vi "6500电流加载及换向回读.vi"(0 "2700 in":refnum<visa-resource-name>, 1 "IT6512C in":refnum<visa-resource-name>, 2 "输入电流":dbl, 3 "Delay Time (s)":dbl=0.5 caption="延迟时间(s)", 5 "error in":errorcluster, 6 "Modbus I/O":refnum<visa-resource-name>) -> (14 "2700 out":refnum<visa-resource-name>, 15 "IT6512C out":refnum<visa-resource-name>, 16 "实际电流":dbl, 19 "error out":errorcluster)   [LabVIEW 2020]
uses:
  <vilib>/Modbus/master/Create Master Instance (Serial).vi
  <instrlib>/Keithley 27XX/Public/Data/Read Single Point.vi
  <vilib>/Modbus/master/Modbus Master.lvclass
  <instrlib>/IT6500/IT6500.lvlib
  <instrlib>/Keithley 27XX/Keithley 27XX.lvlib
panel:
  # "IT6512C 电流加载及换向"
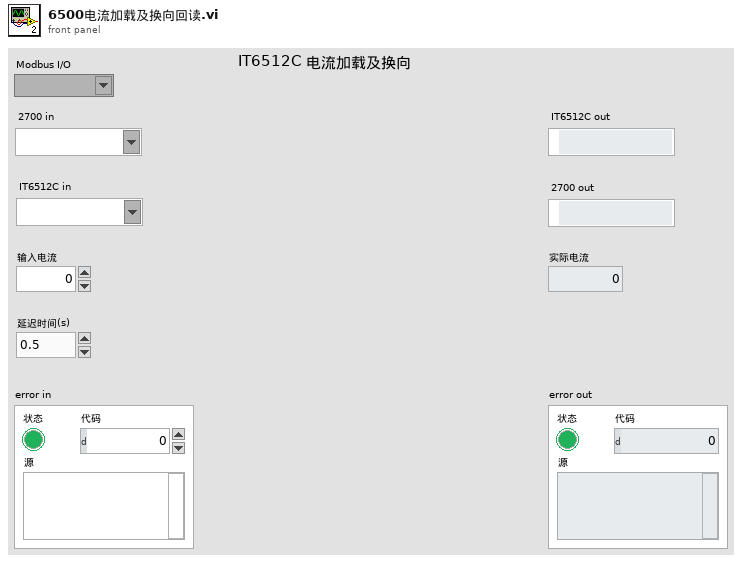
[diagram p1: front panel]
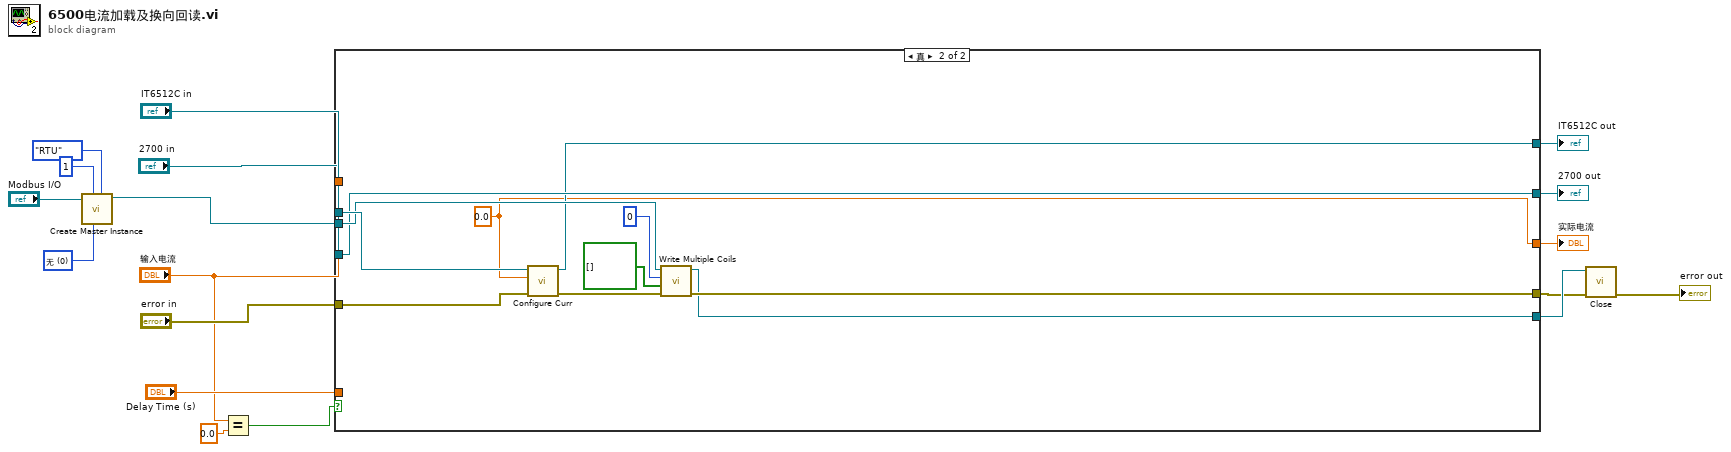
[diagram p0: block diagram]
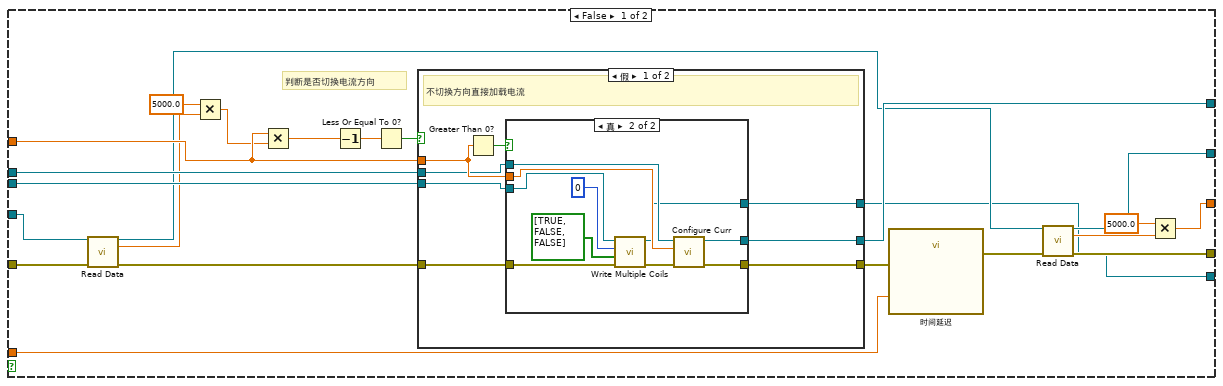
[diagram p2: hidden frame]
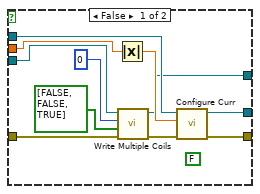
[diagram p3: hidden frame]
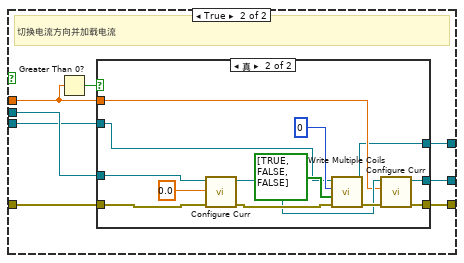
[diagram p4: hidden frame]
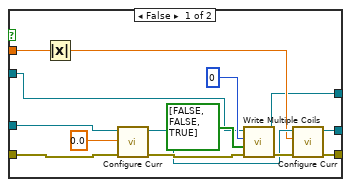
[diagram p5: hidden frame]
diagram:
  w6 = u16 0 items=["无", "奇", "偶"] ("parity (Even)")
  n1 = call-poly <vilib>:"Create Master Instance.vi"("serial type"=enum16{"RTU", "ASCII"}."RTU", "parity (Even)"=w6, "unit ID"=u8 1, "VISA resource name"="Modbus I/O") -> ("serial master instance"=w5:refnum<class "Modbus Master.lvclass">)  [unwired: 6 in, 1 out]
  n2 = Equal?(x="输入电流", y=0.0) -> (x = y?=w10:bool)
  n3 = case shown="真" w10 {
    tunnel: "IT6512C in" -> [w38 w116]
    tunnel: w5 -> [w37 w114]
    tunnel: [w26 w108] -> w3
    tunnel: "Delay Time (s)" -> [w35 _]
    tunnel: "error in" -> [w31 w109]
    tunnel: [w34 w110] -> w15
    tunnel: "2700 in" -> [w32 w111]
    tunnel: [w27 w111] -> w13
    tunnel: "输入电流" -> [w33 _]
    tunnel: [w20 w107] -> w9
    tunnel: [w19 w106] -> w4
    frame False {
      # "判断是否切换电流方向"
      n4 = call-poly <instrlib>:"Read Data.vi"("VISA resource name"=w32, "error in (no error)"=w31) -> ("VISA resource name out"=w29:refnum<visa-resource-name>, "Measurement Data"=w25:dbl, "error out"=w30:errorcluster)  [unwired: 11 in]
      n5 = Multiply(x=5000.0, y=w25) -> (x*y=w23:dbl)
      n6 = Multiply(x=w33, y=w23) -> (x*y=w40:dbl)
      n7 = Decrement(x=w40) -> (x-1=w39:dbl)
      n8 = Less Or Equal To 0?(x=w39) -> (x <= 0?=w41:bool)
      n9 = case shown="假" w41 {
        tunnel: w33 -> [w48 w78]
        tunnel: w30 -> [w45 w73]
        tunnel: w38 -> [w47 w76]
        tunnel: w37 -> [w43 w75]
        tunnel: [w46 w74] -> w36
        tunnel: [w44 w72] -> w34
        tunnel: [w42 w71] -> w19
        frame False {
          # "不切换方向直接加载电流"
          n10 = Greater Than 0?(x=w48) -> (x > 0?=w49:bool)
          n11 = case shown="真" w49 {
            tunnel: w48 -> [w60 w70]
            tunnel: w47 -> [w58 w69]
            tunnel: [w57 w68] -> w46
            tunnel: w45 -> [w54 w62]
            tunnel: [w56 w67] -> w44
            tunnel: w43 -> [w53 w65]
            tunnel: [w50 w61] -> w42
            frame False {
              (unwired) FALSE ("Boolean")
              n12 = Absolute Value(x=w60) -> (abs(x)=w59:dbl)
              n13 = call-dynamic "Write Multiple Coils.vi"("error in (no error)"=w54, "coil values"=bool[] [FALSE, FALSE, TRUE], "starting address"=u16 0, "Modbus master in"=w53) -> ("error out"=w52:errorcluster, "Modbus master out"=w50:refnum<class "Modbus Master.lvclass">)  [unwired: 6 in]
              n14 = call <instrlib>:"Configure Curr.vi"("error in (no error)"=w52, "Curr(0)"=w59, "VISA resource name"=w58) -> ("error out"=w57:errorcluster, "VISA resource name out"=w56:refnum<visa-resource-name>)  [unwired: 7 in]
            }
            frame True {
              n15 = call-dynamic "Write Multiple Coils.vi"("error in (no error)"=w62, "coil values"=bool[] [TRUE, FALSE, FALSE], "starting address"=u16 0, "Modbus master in"=w65) -> ("error out"=w66:errorcluster, "Modbus master out"=w61:refnum<class "Modbus Master.lvclass">)  [unwired: 6 in]
              n16 = call <instrlib>:"Configure Curr.vi"("error in (no error)"=w66, "Curr(0)"=w70, "VISA resource name"=w69) -> ("error out"=w68:errorcluster, "VISA resource name out"=w67:refnum<visa-resource-name>)  [unwired: 7 in]
            }
          }
        }
        frame True {
          # "切换电流方向并加载电流"
          n17 = Greater Than 0?(x=w78) -> (x > 0?=w77:bool)
          n18 = case shown="真" w77 {
            tunnel: w78 -> [w86 w99]
            tunnel: w76 -> [w84 w96]
            tunnel: w75 -> [w83 w98]
            tunnel: [w82 w97] -> w74
            tunnel: w73 -> [w81 w95]
            tunnel: [w80 w94] -> w72
            tunnel: [w79 w93] -> w71
            frame False {
              n19 = Absolute Value(x=w86) -> (abs(x)=w85:dbl)
              n20 = call <instrlib>:"Configure Curr.vi"("error in (no error)"=w81, "Curr(0)"=0.0, "VISA resource name"=w84) -> ("error out"=w89:errorcluster, "VISA resource name out"=w87:refnum<visa-resource-name>)  [unwired: 7 in]
              n21 = call-dynamic "Write Multiple Coils.vi"("error in (no error)"=w89, "coil values"=bool[] [FALSE, FALSE, TRUE], "starting address"=u16 0, "Modbus master in"=w83) -> ("error out"=w88:errorcluster, "Modbus master out"=w79:refnum<class "Modbus Master.lvclass">)  [unwired: 6 in]
              n22 = call <instrlib>:"Configure Curr.vi"("error in (no error)"=w88, "Curr(0)"=w85, "VISA resource name"=w87) -> ("error out"=w82:errorcluster, "VISA resource name out"=w80:refnum<visa-resource-name>)  [unwired: 7 in]
            }
            frame True {
              n23 = call <instrlib>:"Configure Curr.vi"("error in (no error)"=w95, "Curr(0)"=0.0, "VISA resource name"=w96) -> ("error out"=w102:errorcluster, "VISA resource name out"=w100:refnum<visa-resource-name>)  [unwired: 7 in]
              n24 = call-dynamic "Write Multiple Coils.vi"("error in (no error)"=w102, "coil values"=bool[] [TRUE, FALSE, FALSE], "starting address"=u16 0, "Modbus master in"=w98) -> ("error out"=w101:errorcluster, "Modbus master out"=w93:refnum<class "Modbus Master.lvclass">)  [unwired: 6 in]
              n25 = call <instrlib>:"Configure Curr.vi"("error in (no error)"=w101, "Curr(0)"=w99, "VISA resource name"=w100) -> ("error out"=w97:errorcluster, "VISA resource name out"=w94:refnum<visa-resource-name>)  [unwired: 7 in]
            }
          }
        }
      }
      n26 = call "时间延迟"("error in (no error)"=w36, "Delay Time (s)"=w35) -> ("error out"=w28:errorcluster)  [unwired: 9 in]
      n27 = call-poly <instrlib>:"Read Data.vi"("VISA resource name"=w29, "error in (no error)"=w28) -> ("VISA resource name out"=w27:refnum<visa-resource-name>, "Measurement Data"=w22:dbl, "error out"=w26:errorcluster)  [unwired: 11 in]
      n28 = Multiply(x=5000.0, y=w22) -> (x*y=w20:dbl)
    }
    frame True {
      w107 = 0.0 ("Curr(0)")
      n29 = call <instrlib>:"Configure Curr.vi"("error in (no error)"=w109, "Curr(0)"=w107, "VISA resource name"=w116) -> ("error out"=w115:errorcluster, "VISA resource name out"=w110:refnum<visa-resource-name>)  [unwired: 7 in]
      n30 = call-dynamic "Write Multiple Coils.vi"("error in (no error)"=w115, "coil values"=bool[] [], "starting address"=u16 0, "Modbus master in"=w114) -> ("error out"=w108:errorcluster, "Modbus master out"=w106:refnum<class "Modbus Master.lvclass">)  [unwired: 6 in]
    }
  }
  "实际电流" <- w9
  "IT6512C out" <- w15
  "2700 out" <- w13
  n31 = call-dynamic "Close.vi"("error in (no error)"=w3, "Modbus master in"=w4) -> ("error out"=→"error out":errorcluster)  [unwired: 9 in]
